vi "HasSelectionChanged1.vi"(2 "input range":cluster{"x0":dbl, "x1":dbl}, 3 "WFGraph Refnum":refnum<vi>) -> (0 "Selection Changed":bool, 1 "output range":cluster{"x0":dbl, "x1":dbl} {"x1" format="%.2f"; "x0" format="%.2f"})   [LabVIEW 2009]
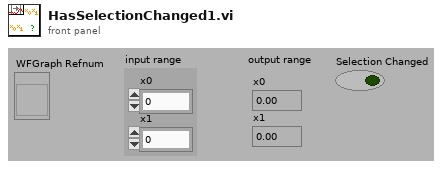
[diagram p1: front panel]
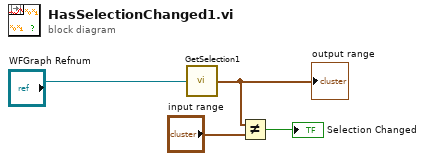
[diagram p0: block diagram]
diagram:
  n1 = call "GetSelection1.vi"("WFGraph Refnum"="WFGraph Refnum") -> ("range"=w2:cluster{"x0":dbl, "x1":dbl})
  "output range" <- w2
  n2 = Not Equal?(x=w2, y="input range") -> (x != y?=→"Selection Changed":bool)
